vi "Update Gyro.vi"(11 "RefNum Name":string) -> ()   [LabVIEW 2013]
uses:
  Gyro Global.vi
panel:
  out "Gyro Index":i32
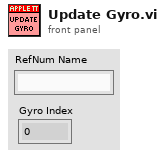
[diagram p1: front panel]
types:
  T1 = typedef "WPI_AnalogChannelDevRef.ctl" = cluster{"DevStatus":errorcluster, "Analog Module":T2, "Analog Channel":T3}
  T2 = typedef "FPGA_TypedefAnalogModule.ctl" = enum16{"Analog Module 1", "Analog Module 2"}
  T3 = typedef "FPGA_AIChannel.ctl" = enum8{"AI 1", "AI 2", "AI 3", "AI 4", "AI 5", "AI 6", "AI 7", "AI 8", "Invalid"}
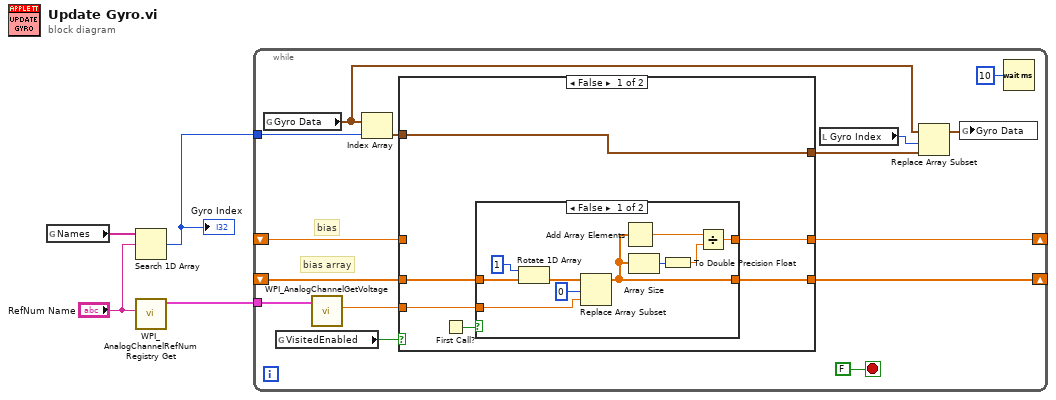
[diagram p0: block diagram]
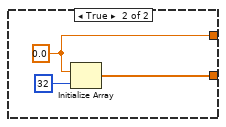
[diagram p2: hidden frame]
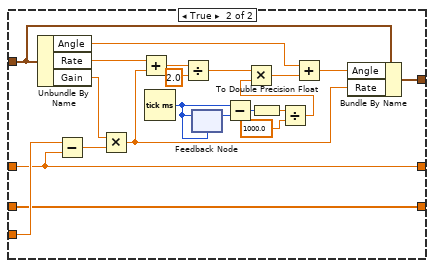
[diagram p3: hidden frame]
diagram:
  n1 = global read "Gyro Global.vi" "Names"() -> (w4:string[])
  n2 = Search 1D Array(1D array=w4, element="RefNum Name") -> (index of element=w1:i32)  [unwired: 1 in]
  "Gyro Index" <- w1
  n3 = call <vilib>:"WPI_AnalogChannelRefNum Registry Get.vi"("refnum name"="RefNum Name") -> ("AIDeviceRef"=w2:T1)  [unwired: 9 in, 1 out]
  n4 = while {
    shift-right: [w17] -> _
    shift-left: _ -> [w16]
    shift-right: [w5] -> _
    shift-left: _ -> [w14]
    tunnel: w2 -> [w13]
    tunnel: w1 -> [w10]
    stop <- FALSE stop-if-true
    # "bias"
    # "bias array"
    n5 = global read "Gyro Global.vi" "Gyro Data"() -> (w6:cluster{"Gain":dbl, "Angle":dbl, "Rate":dbl}[])
    n6 = global read "Gyro Global.vi" "VisitedEnabled"() -> (w15:bool)
    n7 = call <vilib>:"WPI_AnalogChannelGetVoltage.vi"("AIDeviceRef"=w13) -> ("Voltage"=w12:dbl)  [unwired: 8 in, 2 out]
    n8 = Index Array(array=w6, index=w10) -> (element=w11:cluster{"Gain":dbl, "Angle":dbl, "Rate":dbl})
    n9 = case shown="False" w15 {
      tunnel: [w24 w58] -> w17
      tunnel: w16 -> [w23 w58]
      tunnel: [w22 w57] -> w5
      tunnel: w11 -> [w20 w54]
      tunnel: w12 -> [w21 w59]
      tunnel: w14 -> [_ w57]
      tunnel: [w20 w53] -> w9
      frame False {
        n10 = First Call?() -> (First Call?: T/F=w25:bool)
        n11 = case shown="False" w25 {
          tunnel: [w28 w37] -> w24
          tunnel: w23 -> [w35 _]
          tunnel: [w30 w36] -> w22
          tunnel: w21 -> [w27 _]
          frame False {
            n12 = Rotate 1D Array(1:w35, 2:1 ("n")) -> (0:w29:dbl[])
            n13 = Replace Array Subset(array=w29, new element=w27, index=0) -> (w28:dbl[])
            n14 = Add Array Elements(numeric array=w28) -> (sum=w33:dbl)
            n15 = Array Size(array=w28) -> (size(s)=w32:i32)
            n16 = To Double Precision Float(number=w32) -> (double precision float=w31:dbl)
            n17 = Divide(x=w33, y=w31) -> (x/y=w30:dbl)
          }
          frame True {
            w36 = 0.0 ("element")
            n18 = Initialize Array(w36, 32 ("dimension size")) -> (w37:dbl[])
          }
        }
      }
      frame True {
        n19 = Unbundle By Name(w54) -> ("Angle"=w40:dbl, "Rate"=w51:dbl, "Gain"=w55:dbl)
        n20 = Subtract(x=w59, y=w57) -> (x-y=w56:dbl)
        n21 = Multiply(x=w55, y=w56) -> (x*y=w52:dbl)
        n22 = Add(x=w51, y=w52) -> (x+y=w50:dbl)
        n23 = Tick Count (ms)() -> (millisecond timer value=w47:u32)
        n24 = Divide(x=w50, y=2.0) -> (x/y=w48:dbl)
        n25 = feedback-in #1(w47) -> ()
        n26 = feedback #1(w47) -> (w46:u32)
        n27 = Subtract(x=w47, y=w46) -> (x-y=w45:u32)
        n28 = To Double Precision Float(number=w45) -> (double precision float=w44:dbl)
        n29 = Divide(x=w44, y=1000.0) -> (x/y=w42:dbl)
        n30 = Multiply(x=w48, y=w42) -> (x*y=w41:dbl)
        n31 = Add(x=w40, y=w41) -> (x+y=w39:dbl)
        n32 = Bundle By Name(cluster=w54, "Angle"=w39, "Rate"=w52) -> (w53:cluster{"Gain":dbl, "Angle":dbl, "Rate":dbl})
      }
    }
    n33 = local read "Gyro Index"() -> (w8:i32)
    n34 = Replace Array Subset(array=w6, new element=w9, index=w8) -> (w7:cluster{"Gain":dbl, "Angle":dbl, "Rate":dbl}[])
    n35 = global write "Gyro Global.vi" "Gyro Data"(w7) -> ()
    n36 = Wait (ms)(milliseconds to wait=u32 10) -> ()  [unwired: 1 out]
  }
